vi "StopLoop.vi"(7 "Accessibility":T1={"Command"=enum."End", "Error?"=FALSE, "Stop"=FALSE, "StopPomiar"=FALSE, "Name"="", "FilesPath"=path "", "ErrorHandler"={"Threads"=enum."Acquisistion", "ClearError"=FALSE, "Error Out "={"status"=FALSE, "code"=0, "source"=""}, "Error"=FALSE}, "Fs"=0.0}, 11 "error in (no error)":errorcluster) -> (2 "Stop?":bool, 3 "error out":errorcluster)   [LabVIEW 2019]
uses:
  TypeDef/#TypeDef_FromPCtoMR.ctl
  TypeDef/#TypeDef_Command.ctl
  TypeDef/#TypeDef_ErrorHandler_prop.ctl
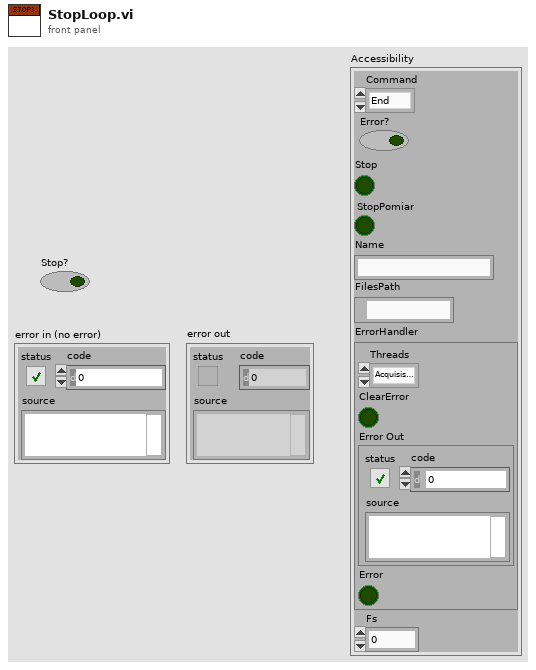
[diagram p1: front panel]
types:
  T1 = typedef "#TypeDef_FromPCtoMR.ctl" = cluster{"Command":T2, "Error?":bool, "Stop":bool, "StopPomiar":bool, "Name":string, "FilesPath":path, "ErrorHandler":T3, "Fs":dbl}
  T2 = typedef "#TypeDef_Command.ctl" = enum16{"Start", "End"}
  T3 = typedef "#TypeDef_ErrorHandler_prop.ctl" = cluster{"Threads":enum16{"Acquisistion", "Data Operation", "Save File"}, "ClearError":bool, "Error Out ":errorcluster, "Error":bool}
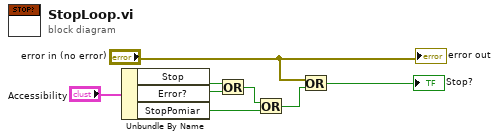
[diagram p0: block diagram]
diagram:
  n1 = Unbundle By Name("Accessibility") -> ("Stop"=w6:bool, "Error?"=w5:bool, "StopPomiar"=w4:bool)
  n2 = Or(x=w6, y=w5) -> (x .or. y?=w3:bool)
  n3 = Or(x=w3, y=w4) -> (x .or. y?=w2:bool)
  n4 = Or(x="error in (no error)", y=w2) -> (x .or. y?=→"Stop?":bool)
  "error out" <- "error in (no error)"
